vi "Create Plugins.vi"(8 "error in (no error)":errorcluster, 11 "Application Data In":T1) -> (0 "error out":errorcluster, 3 "Application Data out":T1)   [LabVIEW 2017, in "DSF Data Viewer.lvlib"]
uses:
  DSF Data Viewer.lvlib
  Main VI/Application Data.ctl
  Core/Engine/Classes/Framework/Framework.lvclass
  Main VI/View Mode.ctl
  Core/Engine/Classes/Framework/Framework.lvclass/Framework.ctl
  ID to Tree Items/Tree Item Type.ctl
  Core/Engine/Classes/Plugin/Plugin.lvclass/Plugin.ctl
  Core/Engine/Classes/Plugin/Plugin.lvclass
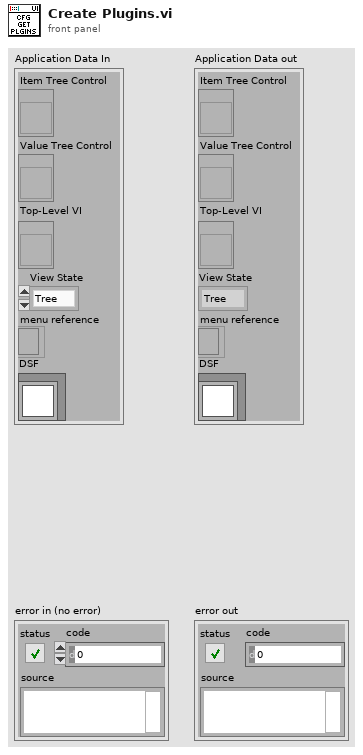
[diagram p1: front panel]
types:
  T1 = typedef "DSF Data Viewer.lvlib/Application Data.ctl" = cluster{"Item Tree Control":refnum<vi>, "Value Tree Control":refnum<vi>, "Top-Level VI":refnum<vi>, "View State":T2, "menu reference":refnum<k9>, "DSF":refnum<class "Framework.lvclass">}
  T2 = typedef "DSF Data Viewer.lvlib/View Mode.ctl" = enum16{"Tree", "List"}
  T3 = typedef "DSF Data Viewer.lvlib/Tree Item Type.ctl" = enum16{"Plugin", "Group", "Transfer", "Buffer", "Channel"}
  T4 = typedef "DSF Data Viewer.lvlib/Tree Item.ctl" = cluster{"Left Cell String":string, "Child Text":string[], "Child Tag":string, "Glyph Index":i32}
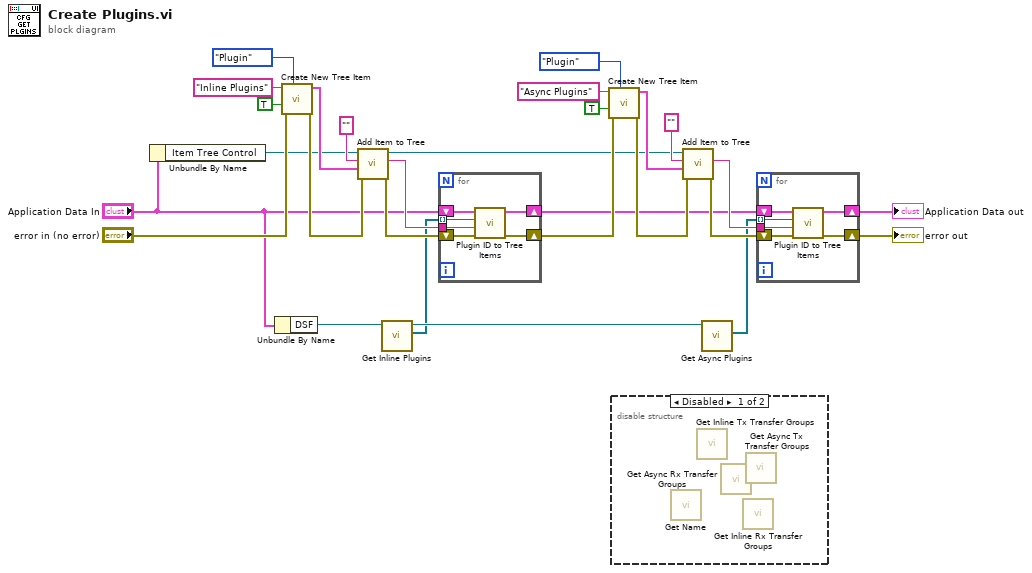
[diagram p0: block diagram]
diagram:
  n1 = Unbundle By Name("Application Data In") -> ("Item Tree Control"=w3:refnum<vi>)
  n2 = Unbundle By Name("Application Data In") -> ("DSF"=w2:refnum<class "Framework.lvclass">)
  n3 = call "Create New Tree Item.vi"("Item Type"=Tree_Item_Type."Plugin", "error in"="error in (no error)", "found?"=TRUE, "Left Cell String"="Inline Plugins") -> ("error out"=w20:errorcluster, "Item"=w22:T4)  [unwired: 6 in]
  n4 = call "Add Item to Tree.vi"("error in (no error)"=w20, "Item"=w22, "parent tag"="", "TreeControl in"=w3) -> ("error out"=w27:errorcluster, "new item tag"=w28:string, "TreeControl out"=w12:refnum<vi>)  [unwired: 5 in]
  n5 = call "Get Inline Plugins.vi"("Framework in"=w2) -> ("Inline Plugins"=w4:refnum<class "Plugin.lvclass">[], "Framework out"=w11:refnum<class "Framework.lvclass">)  [unwired: 9 in]
  n6 = for {
    shift-right: [w33] -> w16
    shift-left: w27 -> [w34]
    tunnel: w4 -> [w31] mode=indexing
    tunnel: w28 -> [w30]
    shift-right: [w29] -> w6
    shift-left: "Application Data In" -> [w32]
    n7 = call "Plugin ID to Tree Items.vi"("error in (no error)"=w34, "parent tag"=w30, "Plugin"=w31, "Application Data in"=w32) -> ("error out"=w33:errorcluster, "Application Data out"=w29:T1)  [unwired: 6 in]
  }
  n8 = call "Create New Tree Item.vi"("Item Type"=Tree_Item_Type."Plugin", "error in"=w16, "found?"=TRUE, "Left Cell String"="Async Plugins") -> ("error out"=w15:errorcluster, "Item"=w13:T4)  [unwired: 6 in]
  n9 = disable-structure shown="Disabled" {
    frame Disabled {
      n10 = call "Get Name.vi"() -> ()  [unwired: 10 in, 2 out]
      n11 = call "Get Inline Tx Transfer Groups.vi"() -> ()  [unwired: 10 in, 2 out]
      n12 = call "Get Async Rx Transfer Groups.vi"() -> ()  [unwired: 10 in, 2 out]
      n13 = call "Get Inline Rx Transfer Groups.vi"() -> ()  [unwired: 10 in, 2 out]
      n14 = call "Get Async Tx Transfer Groups.vi"() -> ()  [unwired: 10 in, 2 out]
    }
    frame Enabled {
    }
  }
  n15 = call "Add Item to Tree.vi"("error in (no error)"=w15, "Item"=w13, "parent tag"="", "TreeControl in"=w12) -> ("error out"=w10:errorcluster, "new item tag"=w7:string)  [unwired: 5 in, 1 out]
  n16 = call "Get Async Plugins.vi"("Framework in"=w11) -> ("Async Plugins"=w5:refnum<class "Plugin.lvclass">[])  [unwired: 9 in, 1 out]
  n17 = for {
    shift-right: [w39] -> w8
    shift-left: w10 -> [w40]
    shift-right: [w37] -> w9
    shift-left: w6 -> [w38]
    tunnel: w7 -> [w36]
    tunnel: w5 -> [w35] mode=indexing
    n18 = call "Plugin ID to Tree Items.vi"("error in (no error)"=w40, "parent tag"=w36, "Plugin"=w35, "Application Data in"=w38) -> ("error out"=w39:errorcluster, "Application Data out"=w37:T1)  [unwired: 6 in]
  }
  "Application Data out" <- w9
  "error out" <- w8
